vi "ProcessButtonPressed.vi"(5 "TimeSinceA":dbl, 6 "Queue in":refnum<queue>, 7 "On Delay Time\nSeconds":dbl, 8 "Time":dbl=-1.0, 9 "ButtonNumber":i32, 10 "ElapsedTime":dbl, 11 "RawButtonInput":bool) -> ()   [LabVIEW 2025]
uses:
  ButtonInfoTypeDef.ctl
  <vilib>/Rock Robotics/WPI/ThirdParty/JAS_Junk/TrajLib/Timer_New.vi
  <vilib>/Utility/semaphor.llb/Obtain Semaphore Reference.vi
  <vilib>/Rock Robotics/WPI/ThirdParty/JAS_Junk/TrajLib/Timer_Reset.vi
  <vilib>/Rock Robotics/WPI/ThirdParty/JAS_Junk/TrajLib/Timer_Start.vi
  <vilib>/Rock Robotics/WPI/ThirdParty/JAS_Junk/TrajLib/Timer_Stop.vi
  <vilib>/Rock Robotics/WPI/ThirdParty/JAS_Junk/TrajLib/Timer_HasPeriodPassedOnce.vi
  Robot Global Data.vi
  <vilib>/Rock Robotics/WPI/ThirdParty/JAS_Junk/TrajLib/Trajectory_Library.lvlib
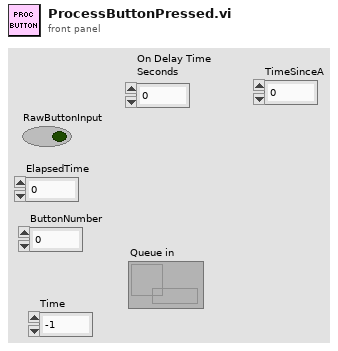
[diagram p1: front panel]
types:
  T1 = typedef "ButtonInfoTypeDef.ctl" = cluster{"ElapsedTime":dbl, "ButtonNumber":i32, "SinceCmdTime":dbl}
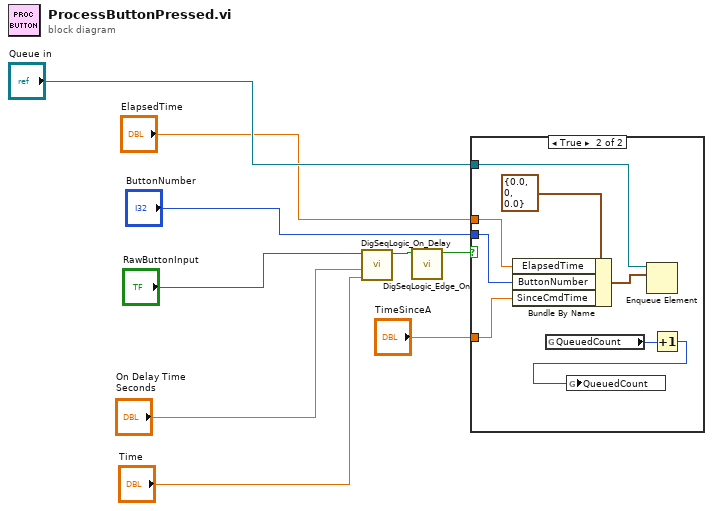
[diagram p0: block diagram]
diagram:
  n1 = call <vilib>:"DigSeqLogic_On_Delay.vi"("Time"="Time", "Delay"="On Delay Time\nSeconds", "Input"="RawButtonInput") -> ("Output"=w5:bool)  [unwired: 7 in, 1 out]
  n2 = call <vilib>:"DigSeqLogic_Edge_On.vi"("Input"=w5) -> ("On Edge"=w6:bool)  [unwired: 10 in]
  n3 = case shown="True" w6 {
    tunnel: "ElapsedTime" -> [_ w16]
    tunnel: "ButtonNumber" -> [_ w15]
    tunnel: "Queue in" -> [_ w14]
    tunnel: "TimeSinceA" -> [_ w10]
    frame False {
    }
    frame True {
      n4 = Bundle By Name(cluster=T1 {"ElapsedTime"=0.0, "ButtonNumber"=0, "SinceCmdTime"=0.0} ("ButtonPressedInfo"), "ElapsedTime"=w16, "ButtonNumber"=w15, "SinceCmdTime"=w10) -> (w13:T1)
      n5 = global read "Robot Global Data.vi" "QueuedCount"() -> (w12:i32)
      n6 = Enqueue Element(queue=w14, element=w13) -> ()  [unwired: 2 in, 3 out]
      n7 = Increment(x=w12) -> (x+1=w11:i32)
      n8 = global write "Robot Global Data.vi" "QueuedCount"(w11) -> ()
    }
  }
